vi "Test VI Print.vi"() -> ()   [LabVIEW 2018, in "Scripts.lvlib"]
uses:
  Scripts.lvlib
panel:
  in  "Images Destination":path=path ""
  in  "VI":path=path ""
  in  "Error In":errorcluster
  out "Error Out":errorcluster
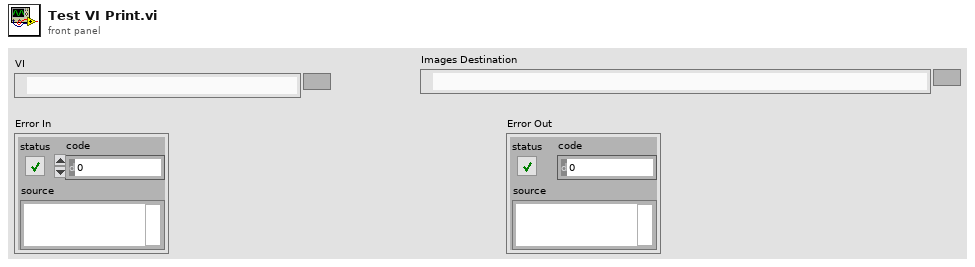
[diagram p1: front panel]
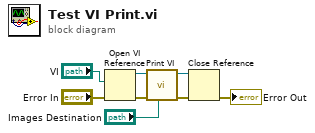
[diagram p0: block diagram]
diagram:
  n1 = Open VI Reference(vi path="VI", error in (no error)="Error In") -> (vi reference=w7:refnum<vi>, error out=w6:errorcluster)  [unwired: 4 in]
  n2 = call "Print VI.vi"("Images Destination"="Images Destination", "Error In"=w6, "VI In"=w7) -> ("Error Out"=w2:errorcluster, "VI Out"=w3:refnum<vi>)  [unwired: 7 in]
  n3 = Close Reference(reference=w3, error in (no error)=w2) -> (error out=→"Error Out":errorcluster)
